vi "AlliGator Phasor References Defined.vi"(9 "Phasor Ratio Reference 2":T2, 10 "Phasor Ratio Reference 1":T2) -> (1 "References Defined":T1(ring))   [LabVIEW 2021, in "AlliGator Phasor Ratio.lvlib"]
doc: "Checks whether all references parameters are defined."
uses:
  Phasor/Phasor (g, s).ctl
  AlliGator Phasor Ratio.lvlib
  Phasor/Phasor.lvlib
panel:
  # "see the AlliGator License on the block diagram (Ctrl+E or Window:Show Block Diagram)"
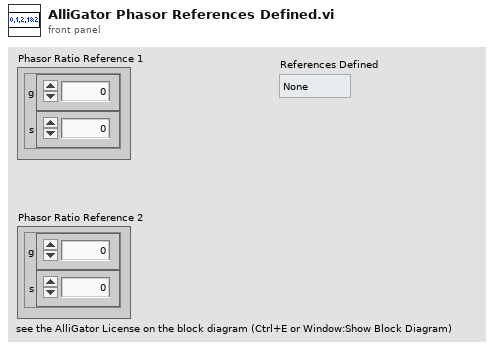
[diagram p1: front panel]
types:
  T1 = enum16{"None", "Reference 1", "Reference 2", "References 1 & 2"}
  T2 = typedef "Phasor.lvlib/Phasor (g, s).ctl" = cluster{"g":dbl, "s":dbl}
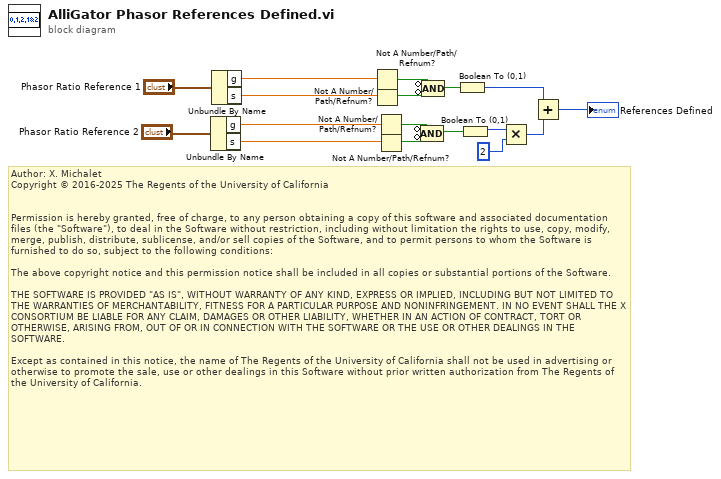
[diagram p0: block diagram]
diagram:
  # "Author: X. Michalet\nCopyright © 2016-2025 The Regents of the University of California\n \n\nPermission is hereby granted, free of charge, to any person obtaining a copy of this software and associated documentation files (the \"Software\"), to deal in the Software without restriction, including without limitation the rights to use, copy, modify, merge, publish, distribute, sublicense, and/or sell copies of the Software, and to permit persons to whom the Software is furnished to do so, subject to the following conditions:\n\nThe above copyright notice and this permission notice shall be included in all copies or substantial portions of the Software.\n\nTHE SOFTWARE IS PROVIDED \"AS IS\", WITHOUT WARRANTY OF ANY KIND, EXPRESS OR IMPLIED, INCLUDING BUT NOT LIMITED TO THE WARRANTIES OF MERCHANTABILITY, FITNESS FOR A PARTICULAR PURPOSE AND NONINFRINGEMENT. IN NO EVENT SHALL THE X CONSORTIUM BE LIABLE FOR ANY CLAIM, DAMAGES OR OTHER LIABILITY, WHETHER IN AN ACTION OF CONTRACT, TORT OR OTHERWISE, ARISING FROM, OUT OF OR IN CONNECTION WITH THE SOFTWARE OR THE USE OR OTHER DEALINGS IN THE SOFTWARE.\n\nExcept as contained in this notice, the name of The Regents of the University of California shall not be used in advertising or otherwise to promote the sale, use or other dealings in this Software without prior written authorization from The Regents of the University of California."
  n1 = Unbundle By Name("Phasor Ratio Reference 2") -> ("g"=w13:dbl, "s"=w12:dbl)
  n2 = Unbundle By Name("Phasor Ratio Reference 1") -> ("g"=w16:dbl, "s"=w15:dbl)
  n3 = Not A Number/Path/Refnum?(number/path/refnum=w16) -> (NaN/Path/Refnum?=w11:bool)
  n4 = Not A Number/Path/Refnum?(number/path/refnum=w15) -> (NaN/Path/Refnum?=w10:bool)
  n5 = Not A Number/Path/Refnum?(number/path/refnum=w13) -> (NaN/Path/Refnum?=w9:bool)
  n6 = Not A Number/Path/Refnum?(number/path/refnum=w12) -> (NaN/Path/Refnum?=w8:bool)
  n7 = Compound Arithmetic op=AND(invert w9, invert w8) -> (w6:bool)
  n8 = Compound Arithmetic op=AND(invert w11, invert w10) -> (w7:bool)
  n9 = Boolean To (0,1)(Boolean=w7) -> (0, 1=w3:i16)
  n10 = Boolean To (0,1)(Boolean=w6) -> (0, 1=w5:i16)
  n11 = Multiply(x=w5, y=i16 2) -> (x*y=w2:i16)
  n12 = Add(x=w3, y=w2) -> (x+y=→"References Defined":i16)
